vi "4021_Module_configure.vi"() -> ()   [LabVIEW 2010]
panel:
  in  "Port Name":string="MainNetwork"
  out "Parameter byte to send":bool[](array[boolean])
  in  "Slew Rate":u8(ring) items=["Instant", "0.0625 V/sec", "0.125 V/sec", "0.250 V/sec", "0.500 V/sec", "1.000 V/sec", "2.000 V/sec", "4.000 V/sec", "8.000 V/sec", "16.000 V/sec", "32.000 V/sec", "64.000 V/sec"]
  in  "Output Range":u16(ring)=2 items=["30   0 to 20mA", "31   4 to 20mA", "32   0 to 10V"]
  in  "Use checksum":bool
  in  "Baud Rate (9600)":u16(ring)=3 items=["1200 bps", "2400 bps", "4800 bps", "9600 bps", "19.2 kbps", "38.4 kbps"]
  in  "Data Format":u8(ring) items=["Engineering Units", "% of FSR", "Hex", "Ohms (4013)"]
  out "Reply":string
  in  "Checksum":bool=TRUE
  out "ConfigStringSent":string
  in  "New Address":u8
  in  "Current Address":u8
  # "0 when INIT*"
  # "Leave off when in INIT*\nOtherwise use checksum"
  # "Can be changed anytime- INIT is not required"
  # "Happy reply starts \"!\"\nUnhappy reply starts \"?\""
  # "Must be in INIT\nto change these"
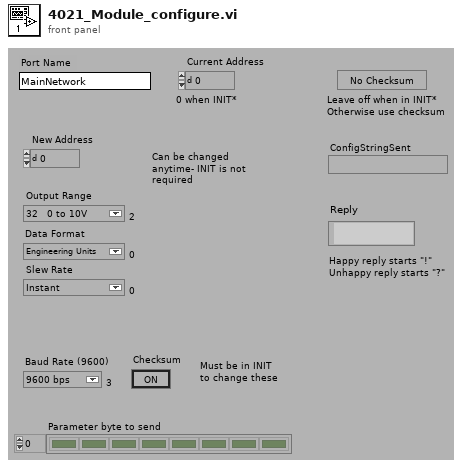
[diagram p1: front panel]
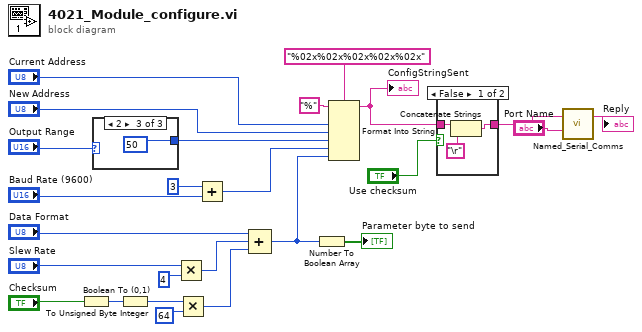
[diagram p0: block diagram]
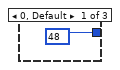
[diagram p2: hidden frame]
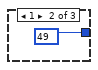
[diagram p3: hidden frame]
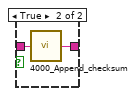
[diagram p4: hidden frame]
diagram:
  n1 = Boolean To (0,1)(Boolean="Checksum") -> (0, 1=w7:i16)
  n2 = case shown="2" "Output Range" {
    tunnel: [48 49 50] -> w13
    frame 0, Default {
    }
    frame 1 {
    }
    frame 2 {
    }
  }
  n3 = To Unsigned Byte Integer(number=w7) -> (unsigned 8bit integer=w4:u8)
  n4 = Multiply(x="Slew Rate", y=u8 4) -> (x*y=w9:u8)
  n5 = Multiply(x=w4, y=u8 64) -> (x*y=w5:u8)
  n6 = Add(x=u16 3, y="Baud Rate (9600)") -> (x+y=w18:u16)
  n7 = Compound Arithmetic op=ADD("Data Format", w9, w5) -> (w3:u8)
  n8 = Number To Boolean Array(number=w3) -> (Boolean array=→"Parameter byte to send":bool[])
  n9 = Format Into String(format string="%02x%02x%02x%02x%02x", initial string="%", "Current Address", "New Address", w13, w18, w3) -> (resulting string=w21:string)  [unwired: 1 in, 1 out]
  "ConfigStringSent" <- w21
  n10 = case shown="False" "Use checksum" {
    tunnel: w21 -> [w31 w33]
    tunnel: [w30 w32] -> w16
    frame False {
      n11 = Concatenate Strings(w31, "\r") -> (w30:string)
    }
    frame True {
      n12 = call "4000_Append_checksum.vi"("ADAM command"=w33) -> ("ADAM string to send"=w32:string)
    }
  }
  n13 = call "Named_Serial_Comms.vi"("Write String"=w16, "Port Name"="Port Name") -> ("Read"=→"Reply":string)  [unwired: 10 in, 3 out]
